vi "Motion_Gantry Check Position.vi"(7 "Tolerance (0.1)":dbl=0.1, 8 "error in (no error)":errorcluster, 10 "Gantry Move Data":T1 {"Z-Position" format="%_7g"; "Y-Position" format="%_7g"; "X-Position" format="%_7g"; "Gantry Velocity" format="%_7g"; "Gantry Accel/Decel" format="%_7g"}, 11 "TCP Connection Refnum":refnum<k5>) -> (0 "error out":errorcluster, 2 "In Position?":bool, 3 "TCP Connection Refnum (dup)":refnum<k5>)   [LabVIEW 2010]
uses:
  Motion_Gantry Position.ctl
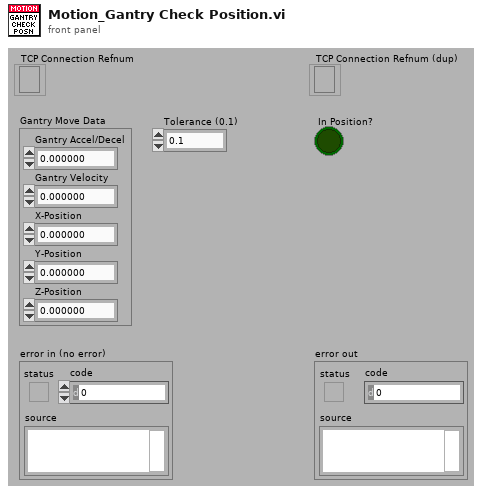
[diagram p1: front panel]
types:
  T1 = typedef "Motion_Gantry Position.ctl" = cluster{"Gantry Accel/Decel":dbl, "Gantry Velocity":dbl, "X-Position":dbl, "Y-Position":dbl, "Z-Position":dbl}
  T2 = cluster{"X-Position":dbl, "Y-Position":dbl, "Z-Position":dbl}
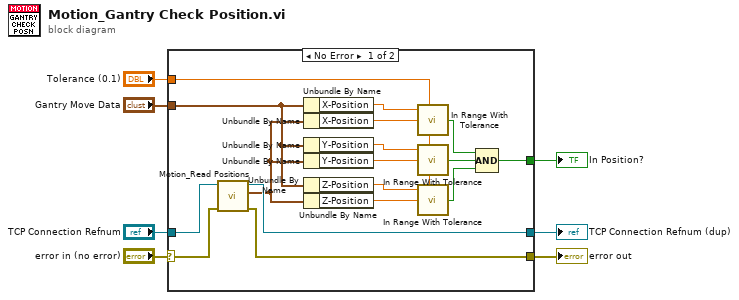
[diagram p0: block diagram]
diagram:
  n1 = case shown="No Error" "error in (no error)" {
    selector: "error in (no error)" -> [w8 w26]
    tunnel: "TCP Connection Refnum" -> [w24 w25]
    tunnel: [w23 w26] -> w6
    tunnel: "Gantry Move Data" -> [w22 _]
    tunnel: [w21 w25] -> w4
    tunnel: [w20 _] -> w3
    tunnel: "Tolerance (0.1)" -> [w11 _]
    frame No Error {
      n2 = call "Motion_Read Positions.vi"("error in"=w8, "TCP Connection Refnum in"=w24) -> ("error out"=w23:errorcluster, "Gantry Position"=w17:T2, "TCP Connection Refnum (dup)"=w21:refnum<k5>)  [unwired: 4 in, 3 out]
      n3 = Unbundle By Name(w22) -> ("X-Position"=w10:dbl)
      n4 = Unbundle By Name(w17) -> ("X-Position"=w9:dbl)
      n5 = Unbundle By Name(w22) -> ("Y-Position"=w15:dbl)
      n6 = Unbundle By Name(w17) -> ("Y-Position"=w19:dbl)
      n7 = Unbundle By Name(w22) -> ("Z-Position"=w16:dbl)
      n8 = Unbundle By Name(w17) -> ("Z-Position"=w18:dbl)
      n9 = call "In Range With Tolerance.vi"("Center"=w10, "Tolerance"=w11, "Value"=w9) -> ("In-Range"=w14:bool)  [unwired: 2 in]
      n10 = call "In Range With Tolerance.vi"("Center"=w15, "Tolerance"=w11, "Value"=w19) -> ("In-Range"=w13:bool)  [unwired: 2 in]
      n11 = call "In Range With Tolerance.vi"("Center"=w16, "Tolerance"=w11, "Value"=w18) -> ("In-Range"=w12:bool)  [unwired: 2 in]
      n12 = Compound Arithmetic op=AND(w14, w13, w12) -> (w20:bool)
    }
    frame Error {
    }
  }
  "error out" <- w6
  "TCP Connection Refnum (dup)" <- w4
  "In Position?" <- w3
